vi "test_PipelineResult_Encode_and_decode.vi"() -> ()   [LabVIEW 2019]
uses:
  <vilib>/Rock Robotics/WPI/ThirdParty/PhotonVisionLib/PhotonVisionLib.lvlib
  <vilib>/Rock Robotics/WPI/ThirdParty/PhotonVisionLib/TypeDef/TargetCornerType.ctl
  <vilib>/Rock Robotics/WPI/ThirdParty/PhotonVisionLib/TypeDef/PhotonTrackedTargetType.ctl
  <vilib>/Rock Robotics/WPI/ThirdParty/PhotonVisionLib/TypeDef/PhotonPipelineResultType.ctl
  <vilib>/Rock Robotics/WPI/ThirdParty/JAS_Junk/TrajLib/TypeDef/TRANSLATION3D.ctl
  <vilib>/Rock Robotics/WPI/ThirdParty/JAS_Junk/TrajLib/Trajectory_Library.lvlib
  <vilib>/Rock Robotics/WPI/ThirdParty/JAS_Junk/TrajLib/TypeDef/QUATERNION.ctl
  <vilib>/Rock Robotics/WPI/ThirdParty/JAS_Junk/TrajLib/TypeDef/ROTATION3D.ctl
  <vilib>/Rock Robotics/WPI/ThirdParty/JAS_Junk/TrajLib/TypeDef/TRANSFORM3D.ctl
panel:
  in  "DetectedCorners 2":T1[](array[typedef])
  in  "DetectedCorners":T1[](array[typedef])
  in  "Fiducial Id 2":i32
  in  "AltCameraToTarget 2":T2={"TRANSLATION3D"={"X"=0.0, "Y"=0.0, "Z"=0.0}, "ROTATION3D"={"Q_quaternion"={"R"=1.0, "V"=[0.0, 0.0, 0.0]}}, "XF"=FALSE} {"TRANSLATION3D"."Z" format="%14.3f"; "TRANSLATION3D"."Y" format="%14.3f"; "TRANSLATION3D"."X" format="%14.3f"}
  in  "BestCameraToTarget 2":T2={"TRANSLATION3D"={"X"=0.0, "Y"=0.0, "Z"=0.0}, "ROTATION3D"={"Q_quaternion"={"R"=1.0, "V"=[0.0, 0.0, 0.0]}}, "XF"=FALSE} {"TRANSLATION3D"."Z" format="%14.3f"; "TRANSLATION3D"."Y" format="%14.3f"; "TRANSLATION3D"."X" format="%14.3f"}
  in  "Pose Ambiguity 2":dbl
  in  "Pitch 2":dbl
  in  "Area 2":dbl
  in  "Skew 2":dbl
  in  "Yaw 2":dbl
  in  "TargetCorners 2":T1[](array[typedef])=[{"X"=0.0, "Y"=0.0}, {"X"=0.0, "Y"=2.0}, {"X"=2.0, "Y"=0.0}, {"X"=2.0, "Y"=2.0}]
  out "Equal":bool
  in  "Fiducial Id":i32
  in  "AltCameraToTarget":T2={"TRANSLATION3D"={"X"=0.0, "Y"=0.0, "Z"=0.0}, "ROTATION3D"={"Q_quaternion"={"R"=1.0, "V"=[0.0, 0.0, 0.0]}}, "XF"=FALSE} {"TRANSLATION3D"."Z" format="%14.3f"; "TRANSLATION3D"."Y" format="%14.3f"; "TRANSLATION3D"."X" format="%14.3f"}
  in  "BestCameraToTarget":T2={"TRANSLATION3D"={"X"=0.0, "Y"=0.0, "Z"=0.0}, "ROTATION3D"={"Q_quaternion"={"R"=1.0, "V"=[0.0, 0.0, 0.0]}}, "XF"=FALSE} {"TRANSLATION3D"."Z" format="%14.3f"; "TRANSLATION3D"."Y" format="%14.3f"; "TRANSLATION3D"."X" format="%14.3f"}
  in  "Pose Ambiguity":dbl
  in  "Pitch":dbl
  in  "Area":dbl
  in  "Skew":dbl
  in  "Yaw":dbl
  in  "TargetCorners":T1[](array[typedef])=[{"X"=-1.0, "Y"=-1.0}, {"X"=-1.0, "Y"=1.0}, {"X"=1.0, "Y"=-1.0}, {"X"=1.0, "Y"=1.0}]
  in  "Latency_Millis":dbl
  out "Packet_RawData":u8[](array[numeric])
  out "Pipeline In":T6 {"Targets"."AltCameraToTarget"."TRANSLATION3D"."Z" format="%14.3f"; "Targets"."AltCameraToTarget"."TRANSLATION3D"."Y" format="%14.3f"; "Targets"."AltCameraToTarget"."TRANSLATION3D"."X" format="%14.3f"; "Targets"."BestCameraToTarget"."TRANSLATION3D"."Z" format="%14.3f"; "Targets"."BestCameraToTarget"."TRANSLATION3D"."Y" format="%14.3f"; "Targets"."BestCameraToTarget"."TRANSLATION3D"."X" format="%14.3f"}
  out "Pipeline Out":T6 {"Targets"."AltCameraToTarget"."TRANSLATION3D"."Z" format="%14.3f"; "Targets"."AltCameraToTarget"."TRANSLATION3D"."Y" format="%14.3f"; "Targets"."AltCameraToTarget"."TRANSLATION3D"."X" format="%14.3f"; "Targets"."BestCameraToTarget"."TRANSLATION3D"."Z" format="%14.3f"; "Targets"."BestCameraToTarget"."TRANSLATION3D"."Y" format="%14.3f"; "Targets"."BestCameraToTarget"."TRANSLATION3D"."X" format="%14.3f"}
  # "FIRST TARGET"
  # "SECOND TARGET"
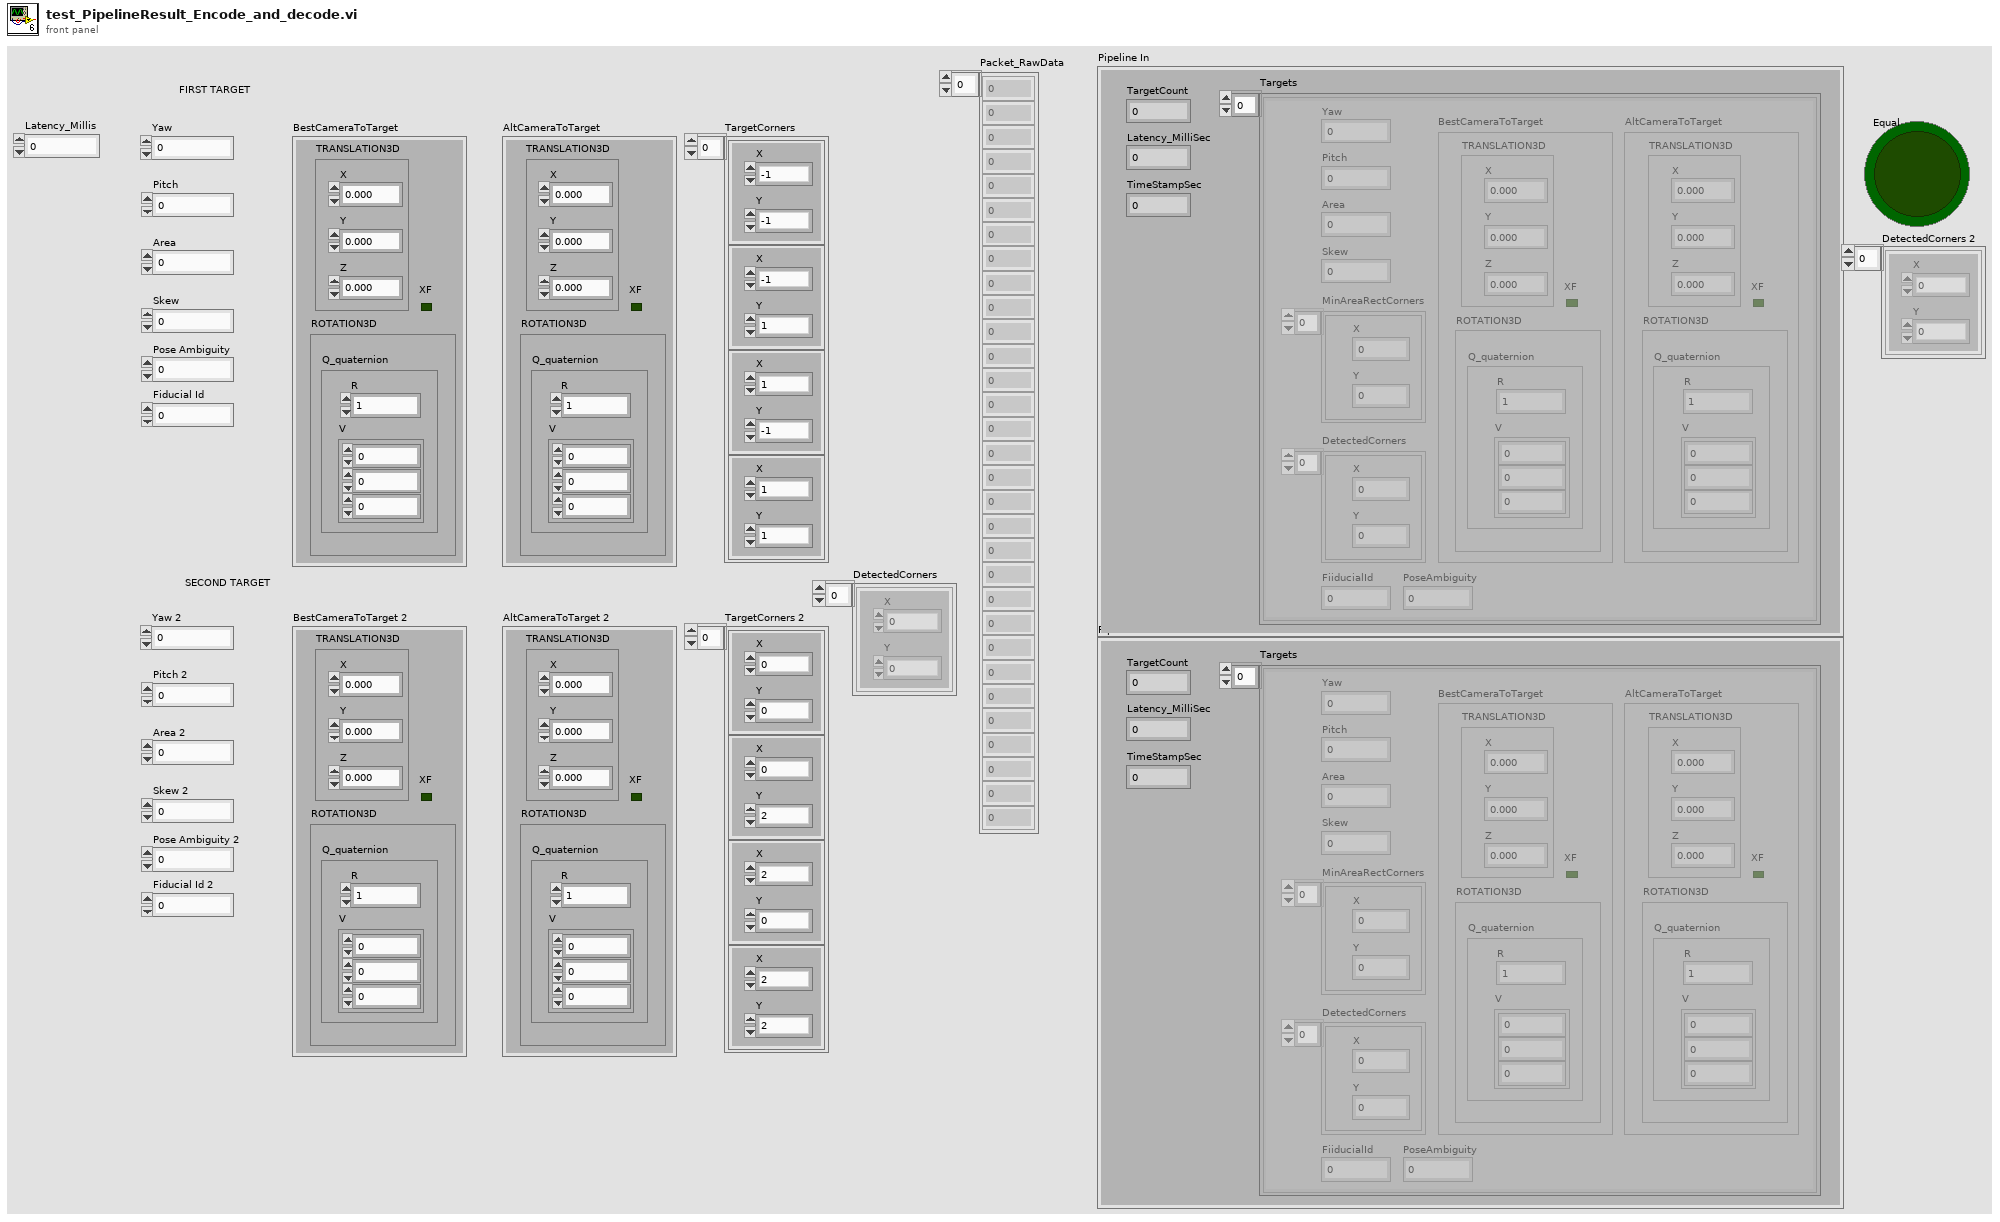
[diagram p1: front panel]
types:
  T1 = typedef "PhotonVisionLib.lvlib/TargetCornerType.ctl" = cluster{"X":dbl, "Y":dbl}
  T2 = typedef "Trajectory_Library.lvlib/TRANSFORM3D.ctl" = cluster{"TRANSLATION3D":T3, "ROTATION3D":T4, "XF":bool}
  T3 = typedef "Trajectory_Library.lvlib/TRANSLATION3D.ctl" = cluster{"X":dbl, "Y":dbl, "Z":dbl}
  T4 = typedef "Trajectory_Library.lvlib/ROTATION3D.ctl" = cluster{"Q_quaternion":T5}
  T5 = typedef "Trajectory_Library.lvlib/QUATERNION.ctl" = cluster{"R":dbl, "V":dbl[]}
  T6 = typedef "PhotonVisionLib.lvlib/PhotonPipelineResultType.ctl" = cluster{"TargetCount":i32, "Latency_MilliSec":dbl, "Targets":T7[], "TimeStampSec":dbl}
  T7 = typedef "PhotonVisionLib.lvlib/PhotonTrackedTargetType.ctl" = cluster{"Yaw":dbl, "Pitch":dbl, "Area":dbl, "Skew":dbl, "MinAreaRectCorners":T1[], "BestCameraToTarget":T2, "FiiducialId":i32, "AltCameraToTarget":T2, "PoseAmbiguity":dbl, "DetectedCorners":T1[]}
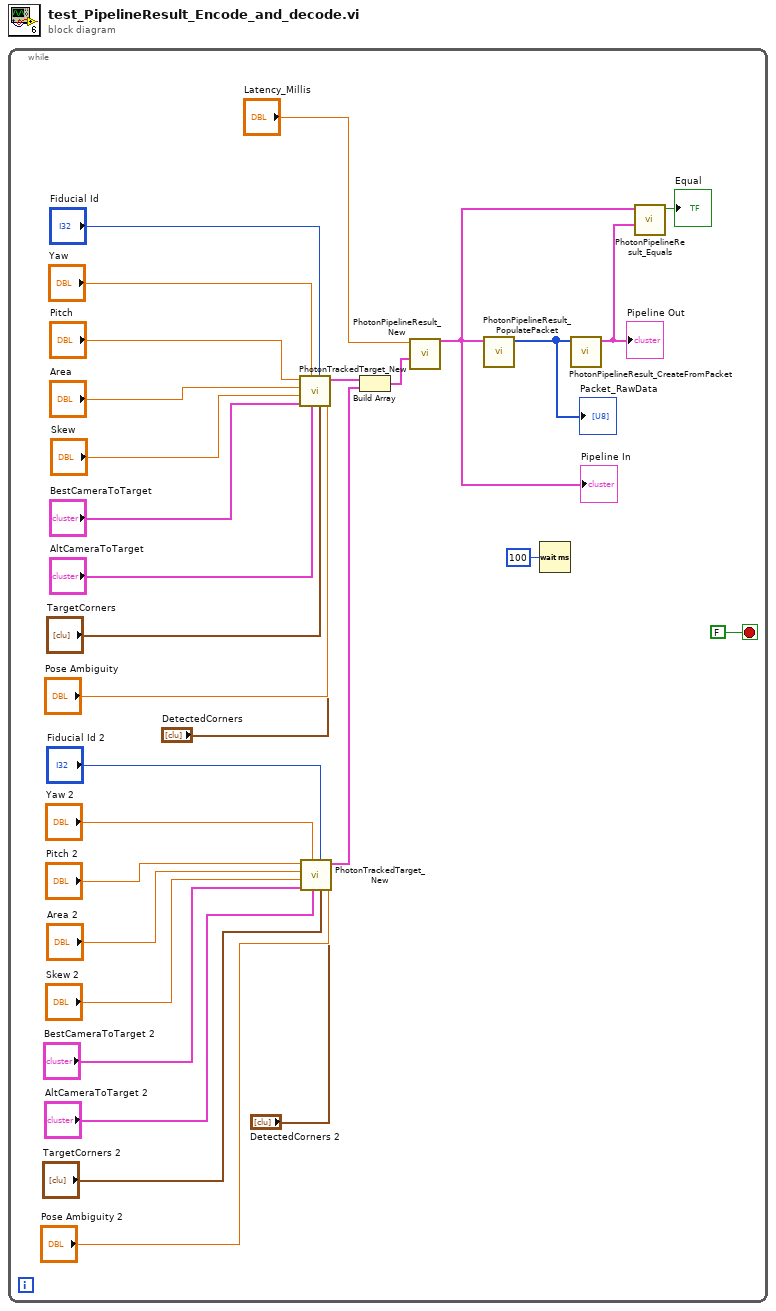
[diagram p0: block diagram]
diagram:
  n1 = while {
    stop <- FALSE stop-if-true
    n2 = call <vilib>:"PhotonTrackedTarget_New.vi"("Pose Ambiguity"="Pose Ambiguity", "DetectedCorners"="DetectedCorners", "MinAreaRectCorners"="TargetCorners", "Fiducial Id"="Fiducial Id", "AltCameraToTarget"="AltCameraToTarget", "Yaw"="Yaw", "BestCameraToTarget"="BestCameraToTarget", "Skew"="Skew", "Area"="Area", "Pitch"="Pitch") -> ("TrackedTarget"=w28:T7)  [unwired: 1 in]
    n3 = call <vilib>:"PhotonTrackedTarget_New.vi"("Pose Ambiguity"="Pose Ambiguity 2", "DetectedCorners"="DetectedCorners 2", "MinAreaRectCorners"="TargetCorners 2", "Fiducial Id"="Fiducial Id 2", "AltCameraToTarget"="AltCameraToTarget 2", "Yaw"="Yaw 2", "BestCameraToTarget"="BestCameraToTarget 2", "Skew"="Skew 2", "Area"="Area 2", "Pitch"="Pitch 2") -> ("TrackedTarget"=w3:T7)  [unwired: 1 in]
    n4 = Build Array(w28, w3) -> (w27:T7[])
    n5 = call <vilib>:"PhotonPipelineResult_New.vi"("TrackedTargets"=w27, "Latency_Millis"="Latency_Millis") -> ("PhotonPipelineResult"=w15:T6)  [unwired: 9 in]
    "Pipeline In" <- w15
    n6 = call <vilib>:"PhotonPipelineResult_PopulatePacket.vi"("PhotonPipelineResult"=w15) -> ("Packet_RawData"=w26:u8[])  [unwired: 10 in]
    "Packet_RawData" <- w26
    n7 = Wait (ms)(milliseconds to wait=u32 100) -> ()  [unwired: 1 out]
    n8 = call <vilib>:"PhotonPipelineResult_CreateFromPacket.vi"("RawData"=w26) -> ("PhotonPipelineResult"=w14:T6)  [unwired: 10 in]
    "Pipeline Out" <- w14
    n9 = call <vilib>:"PhotonPipelineResult_Equals.vi"("Other PhotonPipelineResult"=w14, "PhotonPipelineResult"=w15) -> ("Equal"=→"Equal":bool)  [unwired: 9 in]
  }
